vi "After Launch Init Core.vi"(8 "error in (no error)":errorcluster, 11 "CS++SimMotor in":refnum<class "CS++SimMotor.lvclass">) -> (0 "error out":errorcluster, 3 "CS++SimMotor out":refnum<class "CS++SimMotor.lvclass">)   [LabVIEW 2015, in "CS++SimMotor.lvlib" / "CS++SimMotor.lvclass"]
doc: "Use <b>Pre Launch init.vi</b> method for sanity checks that are supposed to prevent the actor from launching if they fail. Use <B>this</B> method instead to initialize this actor when it has been activated. A corresponding high priority message will become dispatched before the <B>Actor Core.vi</b> is called.\n\n<b>Derived classed should call the parent methode first</b> and their own initialization code after.\n\nRefer also to the ongoing discussion at https://decibel.ni.com/content/message/57394#57394."
uses:
  CS++SimMotor.lvclass
  CS++SimMotor.lvclass/CS++SimMotor.ctl
  <vilib>/ActorFramework/Actor/Actor.lvclass/Actor.ctl
  <vilib>/ActorFramework/Message Enqueuer/Message Enqueuer.lvclass/Message Enqueuer.ctl
  CSPP_Core/Actors/CS++DeviceActor Messages/Reset Device Msg/Reset Device Msg.lvclass/Reset Device Msg.ctl
  <vilib>/ActorFramework/Message Enqueuer/Init from Existing Queue.vi
  <vilib>/ActorFramework/Message Enqueuer/Enqueue.vi
  <vilib>/ActorFramework/Message Priority Queue/Priority Enqueue.vi
  <vilib>/ActorFramework/Message Enqueuer/Message Enqueuer.lvclass
  CSPP_Core/Actors/CS++DeviceActor Messages/Reset Device Msg/Reset Device Msg.lvclass
  CSPP_DeviceBase/CS++Motor/CS++Motor.lvclass
  CSPP_Core/Classes/CS++ProcessVariables/PVConnection/PVConnection.lvclass
  <vilib>/ActorFramework/Actor/Actor.lvclass
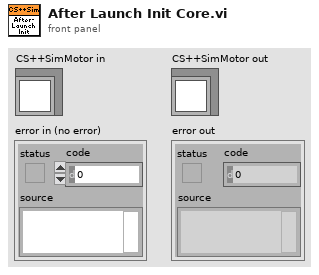
[diagram p1: front panel]
types:
  T1 = cluster{"Read Access":enum8{"Allowed", "Required", "None"}, "Write Access":enum8{"Allowed", "Required", "None"}}
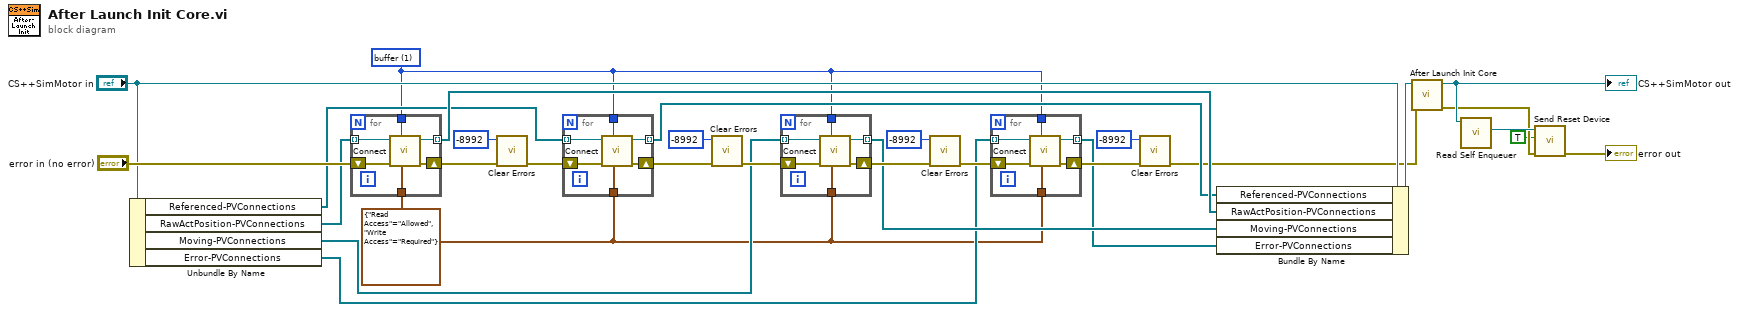
[diagram p0: block diagram]
diagram:
  w9 = u16 1 items=["commit", "buffer"] ("Mode (commit)")
  w6 = T1 {"Read Access"=enum."Allowed", "Write Access"=enum."Required"} ("Access (R/W allowed)")
  n1 = Unbundle By Name("CS++SimMotor in") -> ("Referenced-PVConnections"=w22:refnum<class "PVConnection.lvclass">[], "RawActPosition-PVConnections"=w26:refnum<class "PVConnection.lvclass">[], "Moving-PVConnections"=w15:refnum<class "PVConnection.lvclass">[], "Error-PVConnections"=w8:refnum<class "PVConnection.lvclass">[])
  n2 = for {
    tunnel: w6 -> [w36]
    tunnel: w9 -> [w35]
    tunnel: w26 -> [w32] mode=indexing
    shift-right: [w34] -> w29
    shift-left: "error in (no error)" -> [w33]
    tunnel: [w31] -> w24 mode=indexing
    n3 = call "Connect.vi"("Access (R/W allowed)"=w36, "Mode (buffer)"=w35, "Error In"=w33, "PVConnection in"=w32) -> ("Error Out"=w34:errorcluster, "PVConnection out"=w31:refnum<class "PVConnection.lvclass">)  [unwired: 6 in]
  }
  n4 = call <vilib>:"Clear Errors.vi"("error in (no error)"=w29, "specific error code to clear (0: all)"=-8992) -> ("error out"=w23:errorcluster)  [unwired: 4 in, 1 out]
  n5 = for {
    tunnel: w6 -> [w42]
    tunnel: w9 -> [w41]
    tunnel: w22 -> [w38] mode=indexing
    shift-right: [w40] -> w19
    shift-left: w23 -> [w39]
    tunnel: [w37] -> w21 mode=indexing
    n6 = call "Connect.vi"("Access (R/W allowed)"=w42, "Mode (buffer)"=w41, "Error In"=w39, "PVConnection in"=w38) -> ("Error Out"=w40:errorcluster, "PVConnection out"=w37:refnum<class "PVConnection.lvclass">)  [unwired: 6 in]
  }
  n7 = call <vilib>:"Clear Errors.vi"("error in (no error)"=w19, "specific error code to clear (0: all)"=-8992) -> ("error out"=w16:errorcluster)  [unwired: 4 in, 1 out]
  n8 = for {
    tunnel: w6 -> [w48]
    tunnel: w9 -> [w47]
    tunnel: w15 -> [w44] mode=indexing
    shift-right: [w46] -> w18
    shift-left: w16 -> [w45]
    tunnel: [w43] -> w14 mode=indexing
    n9 = call "Connect.vi"("Access (R/W allowed)"=w48, "Mode (buffer)"=w47, "Error In"=w45, "PVConnection in"=w44) -> ("Error Out"=w46:errorcluster, "PVConnection out"=w43:refnum<class "PVConnection.lvclass">)  [unwired: 6 in]
  }
  n10 = call <vilib>:"Clear Errors.vi"("error in (no error)"=w18, "specific error code to clear (0: all)"=-8992) -> ("error out"=w11:errorcluster)  [unwired: 4 in, 1 out]
  n11 = for {
    tunnel: w6 -> [w54]
    tunnel: w9 -> [w53]
    tunnel: w8 -> [w50] mode=indexing
    shift-right: [w52] -> w12
    shift-left: w11 -> [w51]
    tunnel: [w49] -> w7 mode=indexing
    n12 = call "Connect.vi"("Access (R/W allowed)"=w54, "Mode (buffer)"=w53, "Error In"=w51, "PVConnection in"=w50) -> ("Error Out"=w52:errorcluster, "PVConnection out"=w49:refnum<class "PVConnection.lvclass">)  [unwired: 6 in]
  }
  n13 = call <vilib>:"Clear Errors.vi"("error in (no error)"=w12, "specific error code to clear (0: all)"=-8992) -> ("error out"=w10:errorcluster)  [unwired: 4 in, 1 out]
  n14 = Bundle By Name(cluster="CS++SimMotor in", "Referenced-PVConnections"=w21, "RawActPosition-PVConnections"=w24, "Moving-PVConnections"=w14, "Error-PVConnections"=w7) -> (w25:refnum<class "CS++SimMotor.lvclass">)
  n15 = call-parent "After Launch Init Core.vi"("error in (no error)"=w10, "CS++Motor in"=w25) -> ("error out"=w3:errorcluster, "CS++Motor out"=w5:refnum<class "CS++SimMotor.lvclass">)  [unwired: 8 in]
  "CS++SimMotor out" <- w5
  n16 = call <vilib>:"Read Self Enqueuer.vi"("Actor"=w5) -> ("Self Enqueuer"=w4:refnum<class "Message Enqueuer.lvclass">)  [unwired: 10 in]
  n17 = call "Send Reset Device.vi"("error in (no error)"=w3, "Reset"=TRUE, "Message Enqueuer"=w4) -> ("error out"=→"error out":errorcluster)  [unwired: 7 in, 1 out]
